vi "音乐盒.vi"   [LabVIEW 2018]
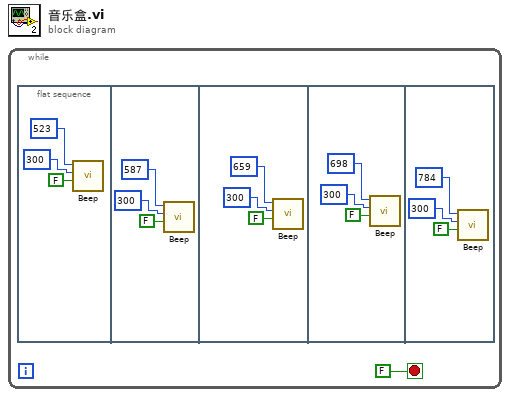
[diagram p0: block diagram]
diagram:
  n1 = while {
    stop <- FALSE stop-if-true
    n2 = flat-sequence {
      frame #0 {
        n3 = call <vilib>:"Beep.vi"("use system alert? (T)"=FALSE, "duration (msec)"=300, "frequency (Hz)"=523) -> ()  [unwired: 9 in]
      }
      frame #1 {
        n4 = call <vilib>:"Beep.vi"("use system alert? (T)"=FALSE, "duration (msec)"=300, "frequency (Hz)"=587) -> ()  [unwired: 9 in]
      }
      frame #2 {
        n5 = call <vilib>:"Beep.vi"("use system alert? (T)"=FALSE, "duration (msec)"=300, "frequency (Hz)"=659) -> ()  [unwired: 9 in]
      }
      frame #3 {
        n6 = call <vilib>:"Beep.vi"("use system alert? (T)"=FALSE, "duration (msec)"=300, "frequency (Hz)"=698) -> ()  [unwired: 9 in]
      }
      frame #4 {
        n7 = call <vilib>:"Beep.vi"("use system alert? (T)"=FALSE, "duration (msec)"=300, "frequency (Hz)"=784) -> ()  [unwired: 9 in]
      }
    }
  }
